vi "set pretomo cubic volume.vi"(8 "error in (no error)":errorcluster, 11 "Tomo in":refnum<class "Tomo.lvclass">) -> (0 "error out":errorcluster, 3 "Tomo out":refnum<class "Tomo.lvclass">)   [LabVIEW 2012, in "Tomo.lvclass"]
uses:
  Tomo.lvclass
  Tomo.lvclass/Tomo.ctl
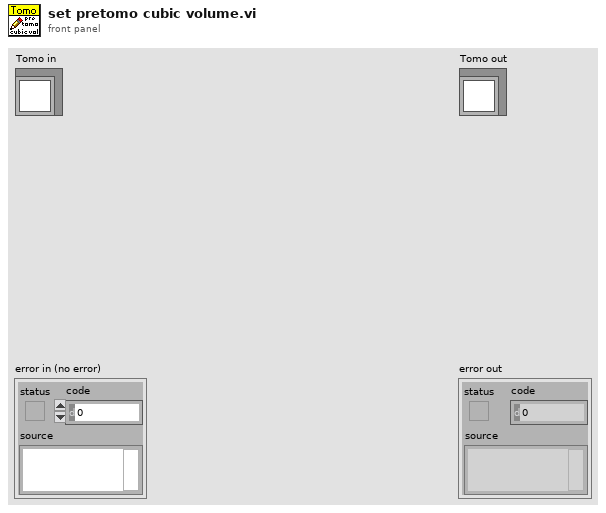
[diagram p1: front panel]
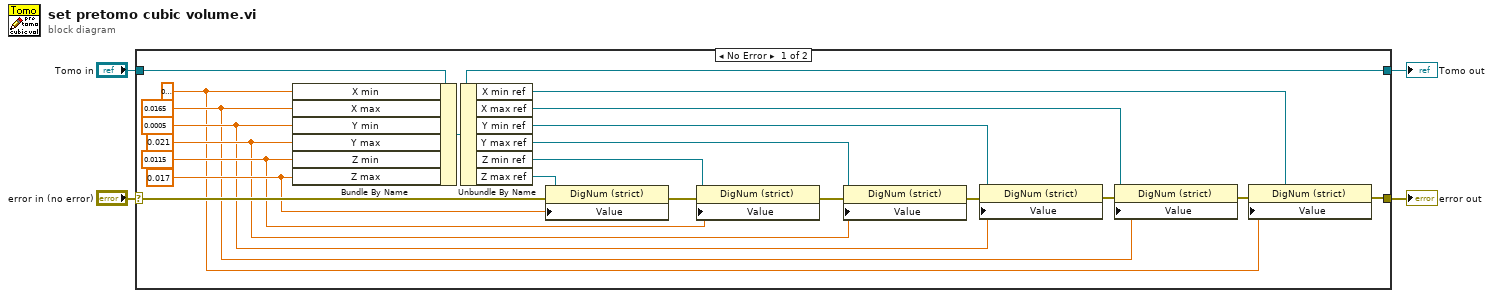
[diagram p0: block diagram]
diagram:
  n1 = case shown="No Error" "error in (no error)" {
    selector: "error in (no error)" -> [w24 w27]
    tunnel: [w18 w27] -> w3
    tunnel: [w23 w26] -> w1
    tunnel: "Tomo in" -> [w25 w26]
    frame No Error {
      w10 = dbl[unit] 0.017 ("settings.coordinates.Z max")
      w9 = dbl[unit] 0.0115 ("settings.coordinates.Z min")
      w8 = dbl[unit] 0.021 ("settings.coordinates.Y max")
      w7 = dbl[unit] 0.0005 ("settings.coordinates.Y min")
      w6 = dbl[unit] 0.0165 ("settings.coordinates.X max")
      w5 = dbl[unit] 0.007 ("settings.coordinates.X min")
      n2 = Bundle By Name(cluster=w25, "X min"=w5, "X max"=w6, "Y min"=w7, "Y max"=w8, "Z min"=w9, "Z max"=w10) -> (w23:refnum<class "Tomo.lvclass">)
      n3 = Unbundle By Name(w23) -> ("X min ref"=w16:refnum<vi>, "X max ref"=w15:refnum<vi>, "Y min ref"=w14:refnum<vi>, "Y max ref"=w13:refnum<vi>, "Z min ref"=w12:refnum<vi>, "Z max ref"=w11:refnum<vi>)
      n4 = property class="DigNum (strict)"(reference=w11, error in=w24, "Value"=w10) -> (error out=w22:errorcluster)  [unwired: 1 out]
      n5 = property class="DigNum (strict)"(reference=w12, error in=w22, "Value"=w9) -> (error out=w21:errorcluster)  [unwired: 1 out]
      n6 = property class="DigNum (strict)"(reference=w13, error in=w21, "Value"=w8) -> (error out=w17:errorcluster)  [unwired: 1 out]
      n7 = property class="DigNum (strict)"(reference=w14, error in=w17, "Value"=w7) -> (error out=w19:errorcluster)  [unwired: 1 out]
      n8 = property class="DigNum (strict)"(reference=w15, error in=w19, "Value"=w6) -> (error out=w20:errorcluster)  [unwired: 1 out]
      n9 = property class="DigNum (strict)"(reference=w16, error in=w20, "Value"=w5) -> (error out=w18:errorcluster)  [unwired: 1 out]
    }
    frame Error {
    }
  }
  "error out" <- w3
  "Tomo out" <- w1
